vi "AuMT8852B Event Status Enable.vi"(5 "Flags (all disabled)":T1, 7 "Set/Get (Set)":enum16{"Set", "Get"}(ring), 8 "error in (no error)":errorcluster, 10 "Value (-1)":i32=-1, 11 "VISA session":refnum<visa-resource-name>) -> (0 "error out":errorcluster, 2 "error code":i32, 3 "VISA session out":refnum<visa-resource-name>, 4 "Flags out":T1, 6 "Value out":i32)   [LabVIEW 2017]
doc: "Anritsu MT8852B Bluetooth Tester\n\nIndicates which bits of the IEE-488.2 standard Event Status Register will cause a Service Request (SRQ). The value can be written as an integer (0-255), or as a cluster of flags.\n\nBit 7 (most significant bit) - Power on - this bit is set on power up of the device only and cleared if the instrument is reset or receives a *CLS command. This bit only indicates that a power on has occurred.\n\nBit 6 - User reqest - unused.\n\nBit 5 - Command error - received an unrecognized command.\n\nBit 4 - Execution error - could not execute a command. For example, a parameter is out of the allowable range.\n\nBit 3 - Device dependent error - the specific error can be found by using the ERRLST command.\n\nBit 2 - Query error.\n\nBit 1 - Request control. GPIB controllers only.\n\nBit 0 (least significant bit) - Operation complete. When a program message that includes the *OPC command has been completed and the GPIB interface is idle with any responses read out of the output buffer, this bit is set. For example, if the last command in a configuration sequence is *OPC, the OPC bit in the event status register will be set when that configuration list has been completed.\n\nINPUTS\nSet/Get - whether the values are being written to or read from the instrument.\nFlags - individual values to assign to the register.\nValue - integer value (0-255) to be written to the register. Leave this input unwired if you are using the Flags input.\n\nOUTPUTS\nFlags out - value of each bit in the register.\nValue out - integer value (0-255) of the register."
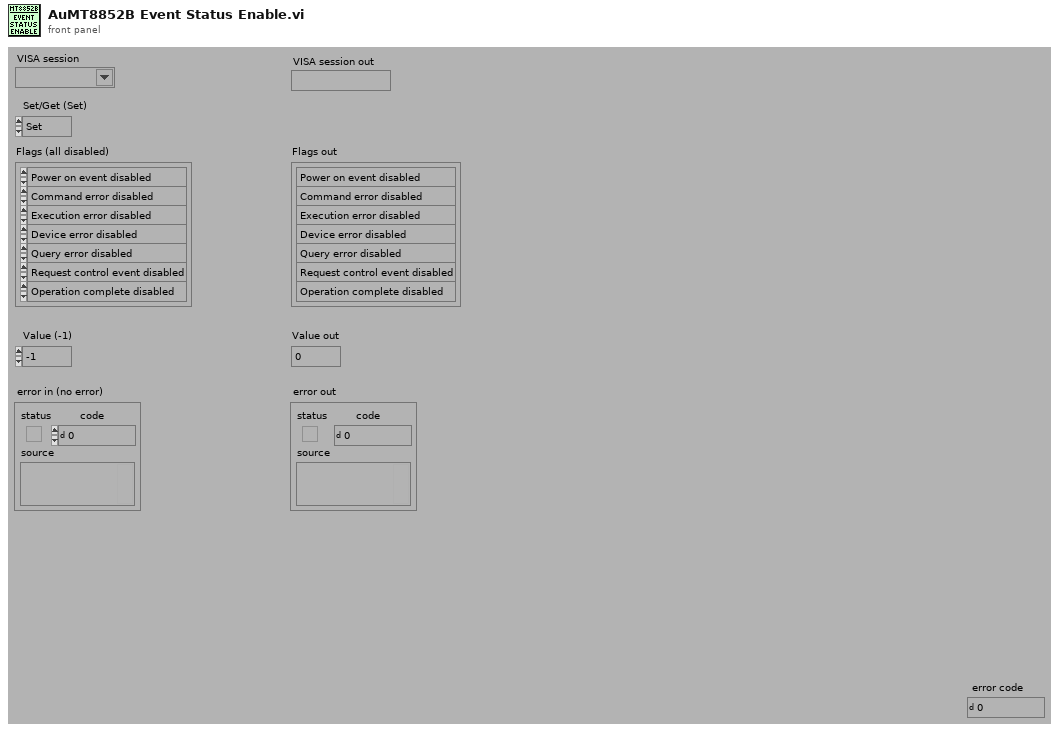
[diagram p1: front panel]
types:
  T1 = cluster{"Power on":enum16{"Power on event disabled", "Power on event enabled"}, "Command":enum16{"Command error disabled", "Command error enabled"}, "Execution":enum16{"Execution error disabled", "Execution error enabled"}, "Device":enum16{"Device error disabled", "Device error enabled"}, "Query":enum16{"Query error disabled", "Query error enabled"}, "Request control":enum16{"Request control event disabled", "Request control event enabled"}, "Operation":enum16{"Operation complete disabled", "Operation complete enabled"}}
  T2 = enum16{"Simulate", "Range check", "Cache", "Query instrument status"}
  T3 = cluster{"[0]":i16, "[1]":i16, "[2]":i16, "[3]":i16, "[4]":i16, "[5]":i16, "[6]":i16, "[7]":i16}
  T4 = enum16{"Operation complete disabled", "Operation complete enabled"}
  T5 = enum16{"Request control event disabled", "Request control event enabled"}
  T6 = enum16{"Query error disabled", "Query error enabled"}
  T7 = enum16{"Device error disabled", "Device error enabled"}
  T8 = enum16{"Execution error disabled", "Execution error enabled"}
  T9 = enum16{"Command error disabled", "Command error enabled"}
  T10 = enum16{"Power on event disabled", "Power on event enabled"}
  T11 = cluster{bool, bool, bool, bool, bool, bool, bool, bool}
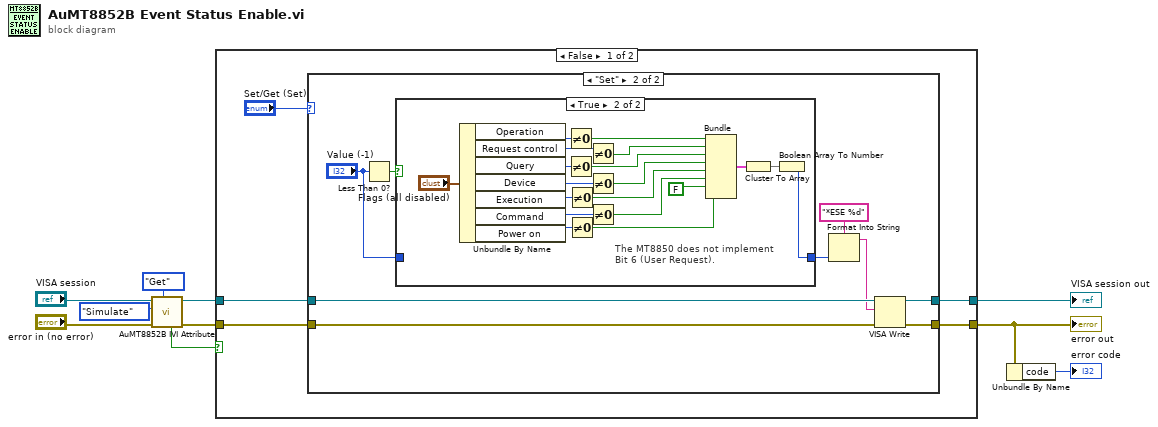
[diagram p0: block diagram]
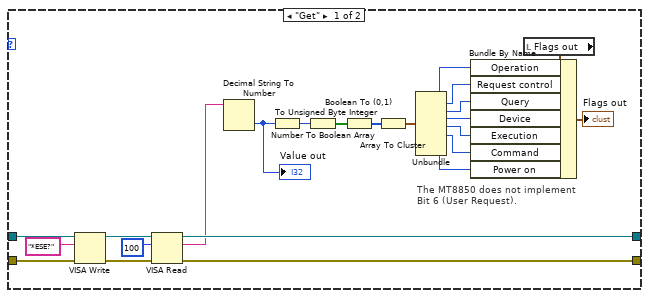
[diagram p2: hidden frame]
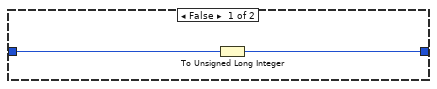
[diagram p3: hidden frame]
diagram:
  n1 = call <instrlib>:"AuMT8852B IVI Attribute.vi"("Set/Get (Set)"=enum16{"Set", "Get"}."Get", "error in (no error)"="error in (no error)", "Flag (Simulate)"=T2."Simulate", "VISA session"="VISA session") -> ("error out"=w6:errorcluster, "VISA session out"=w7:refnum<visa-resource-name>, "Value out"=w3:bool)  [unwired: 5 in]
  n2 = case shown="False" w3 {
    tunnel: [w12 w69] -> w1
    tunnel: [w13 w70] -> w8
    tunnel: w7 -> [w15 w70]
    tunnel: w6 -> [w14 w69]
    frame False {
      n3 = case shown="\"Set\"" "Set/Get (Set)" {
        tunnel: w15 -> [w38 w47]
        tunnel: w14 -> [w37 w46]
        tunnel: [w33 w43] -> w13
        tunnel: [w32 w42] -> w12
        frame "Get" {
          # "The MT8850 does not implement\nBit 6 (User Request)."
          n4 = VISA Write(VISA resource name=w38, write buffer="*ESE?" ("write buffer (\"\")"), error in (no error)=w37) -> (VISA resource name out=w35:refnum<visa-resource-name>, error out=w34:errorcluster)  [unwired: 1 out]
          n5 = VISA Read(VISA resource name=w35, byte count=u32 100 ("byte count (0)"), error in (no error)=w34) -> (VISA resource name out=w33:refnum<visa-resource-name>, read buffer=w30:string, error out=w32:errorcluster)  [unwired: 1 out]
          n6 = Decimal String To Number(string=w30) -> (number=w16:i32)  [unwired: 2 in, 1 out]
          "Value out" <- w16
          n7 = To Unsigned Byte Integer(number=w16) -> (unsigned 8bit integer=w17:u8)
          n8 = Number To Boolean Array(number=w17) -> (Boolean array=w18:bool[])
          n9 = Boolean To (0,1)(Boolean=w18) -> (0, 1=w19:i16[])
          n10 = Array To Cluster(array=w19) -> (cluster=w27:T3)
          n11 = Unbundle(w27) -> ("[0]"=w20:i16, "[1]"=w21:i16, "[2]"=w22:i16, "[3]"=w23:i16, "[4]"=w24:i16, "[5]"=w25:i16, "[7]"=w26:i16)  [unwired: 1 out]
          n12 = local read "Flags out"() -> (w28:T1)
          n13 = Bundle By Name(cluster=w28, "Operation"=w20, "Request control"=w21, "Query"=w22, "Device"=w23, "Execution"=w24, "Command"=w25, "Power on"=w26) -> (→"Flags out":T1)
        }
        frame "Set" {
          n14 = Less Than 0?(x="Value (-1)") -> (x < 0?=w40:bool)
          n15 = case shown="True" w40 {
            tunnel: [w48 w56] -> w44
            tunnel: "Value (-1)" -> [w49 _]
            frame False {
              n16 = To Unsigned Long Integer(number=w49) -> (unsigned 32bit integer=w48:u32)
            }
            frame True {
              # "The MT8850 does not implement\nBit 6 (User Request)."
              n17 = Unbundle By Name("Flags (all disabled)") -> ("Operation"=w67:T4, "Request control"=w55:T5, "Query"=w54:T6, "Device"=w53:T7, "Execution"=w52:T8, "Command"=w51:T9, "Power on"=w50:T10)
              n18 = Not Equal To 0?(x=w67) -> (x != 0?=w66:bool)
              n19 = Not Equal To 0?(x=w54) -> (x != 0?=w64:bool)
              n20 = Not Equal To 0?(x=w52) -> (x != 0?=w62:bool)
              n21 = Not Equal To 0?(x=w50) -> (x != 0?=w59:bool)
              n22 = Not Equal To 0?(x=w55) -> (x != 0?=w65:bool)
              n23 = Not Equal To 0?(x=w53) -> (x != 0?=w63:bool)
              n24 = Not Equal To 0?(x=w51) -> (x != 0?=w61:bool)
              n25 = Bundle(w66, w65, w64, w63, w62, w61, FALSE, w59) -> (w58:T11)  [unwired: 1 in]
              n26 = Cluster To Array(cluster=w58) -> (array=w57:bool[])
              n27 = Boolean Array To Number(Boolean array=w57) -> (number=w56:u32)
            }
          }
          n28 = Format Into String(format string="*ESE %d" ("Format String"), w44) -> (resulting string=w41:string)  [unwired: 2 in, 1 out]
          n29 = VISA Write(VISA resource name=w47, write buffer=w41, error in (no error)=w46) -> (VISA resource name out=w43:refnum<visa-resource-name>, error out=w42:errorcluster)  [unwired: 1 out]
        }
      }
    }
    frame True {
    }
  }
  "error out" <- w1
  "VISA session out" <- w8
  n30 = Unbundle By Name(w1) -> ("code"=→"error code":i32)
